vi "get write location linear fit.vi"(7 "use line and frame numbers":bool, 9 "xyz order":bool, 10 "current volume":T1={"min x"=-1638, "deltaX"=41.0, "num x"=79, "max x"=1601, "min y"=-1638, "deltaY"=41.0, "num y"=80, "max y"=1642, "num z"=30, "num voxels"=189600, "voxels read"=0, "volume num"=0}, 11 "line":T2) -> (3 "3D write locations":u32[](array[numeric]))   [LabVIEW 2010]
uses:
  line_info.ctl
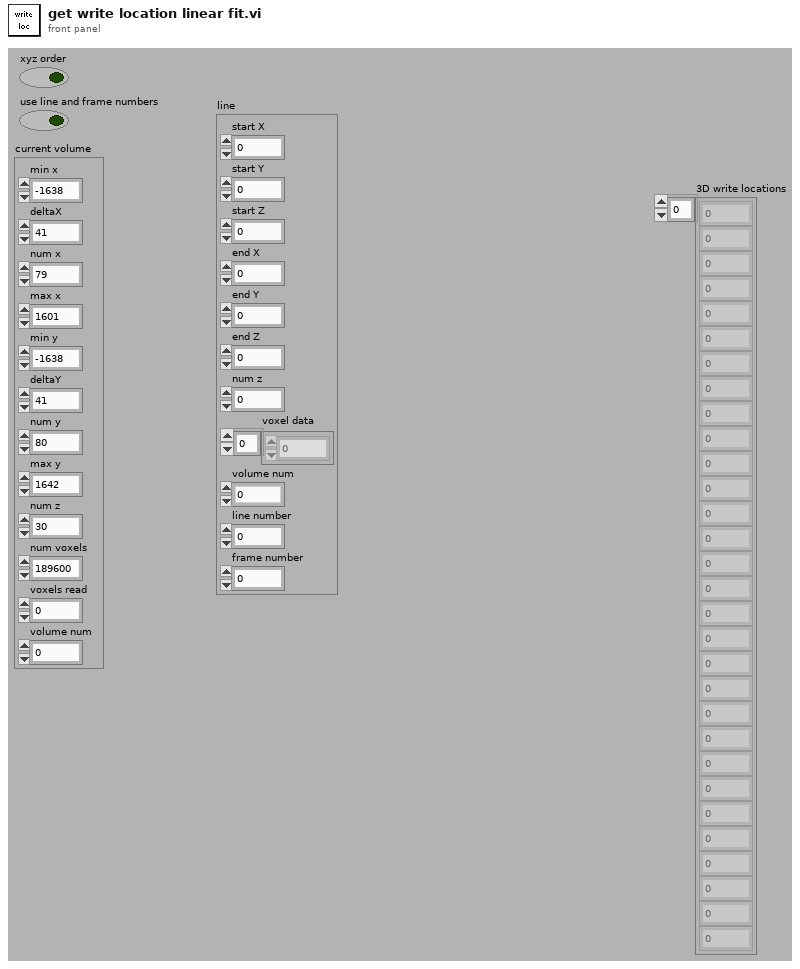
[diagram p1: front panel]
types:
  T1 = cluster{"min x":i16, "deltaX":dbl, "num x":u32, "max x":i16, "min y":i16, "deltaY":dbl, "num y":u32, "max y":i16, "num z":u32, "num voxels":u32, "voxels read":u32, "volume num":u32}
  T2 = typedef "line_info.ctl" = cluster{"start X":i16, "start Y":i16, "start Z":i16, "end X":i16, "end Y":i16, "end Z":i16, "num z":u8, "voxel data":u32[], "volume num":u32, "line number":u16, "frame number":u16}
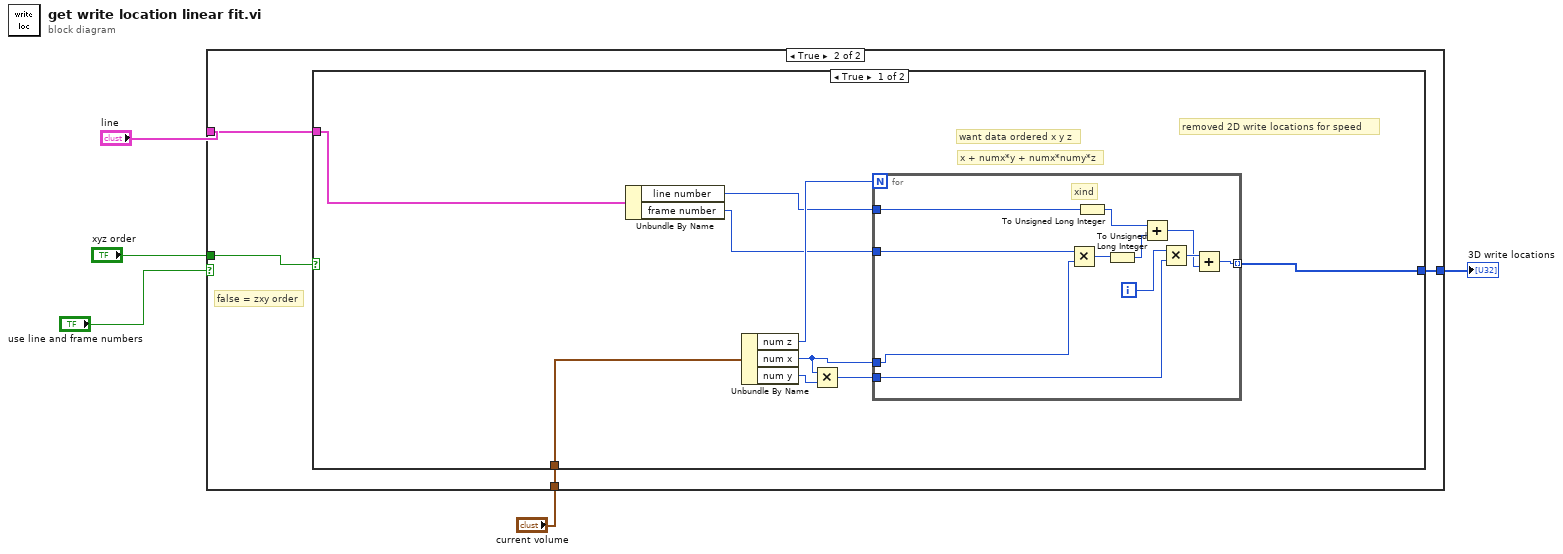
[diagram p0: block diagram]
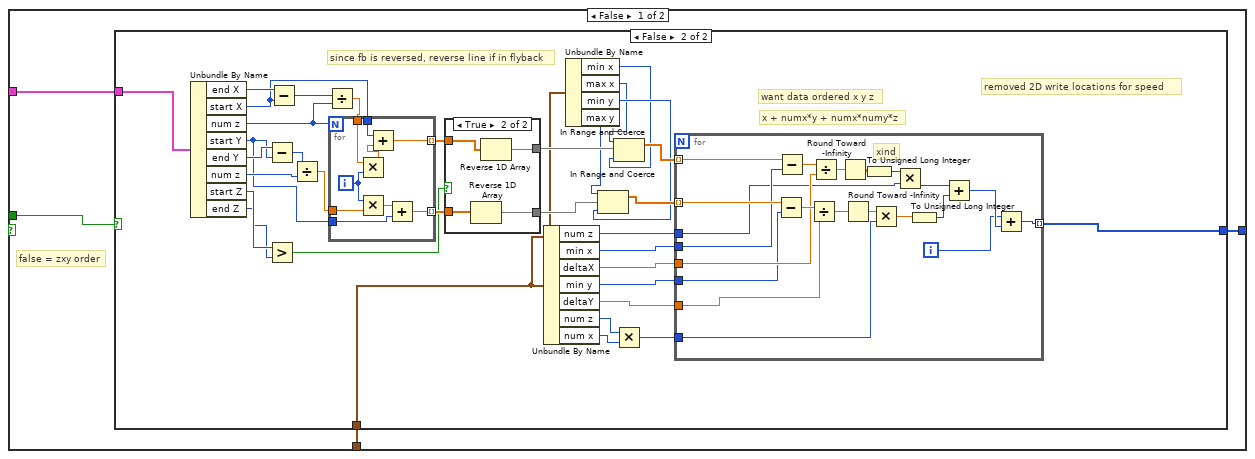
[diagram p2: hidden frame]
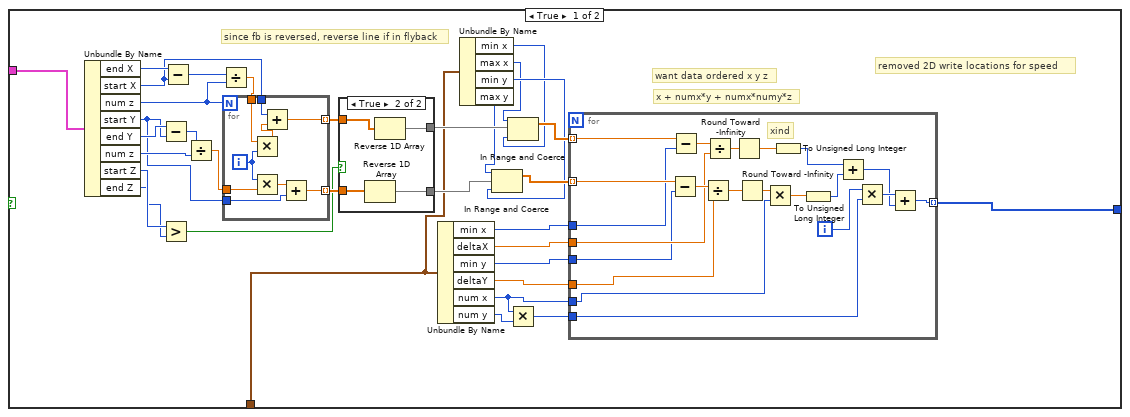
[diagram p3: hidden frame]
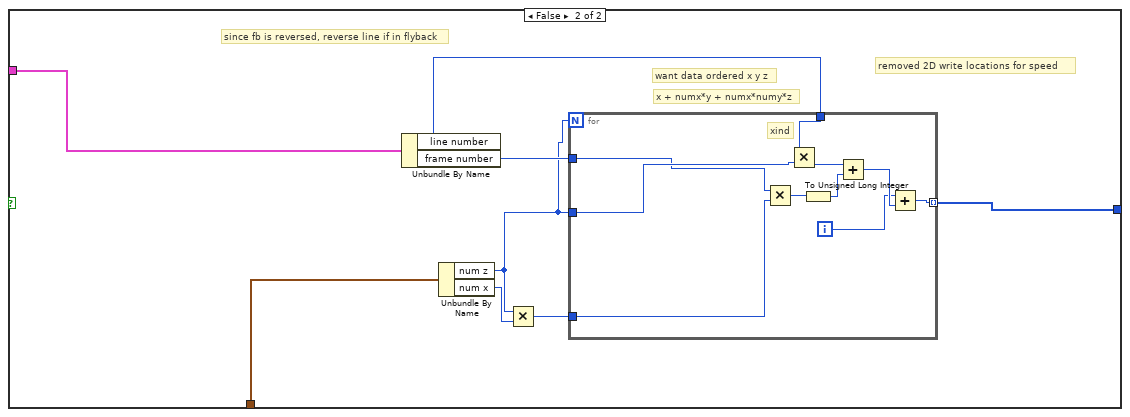
[diagram p6: hidden frame]
diagram:
  n1 = case shown="True" "use line and frame numbers" {
    tunnel: "line" -> [w9 w152]
    tunnel: "xyz order" -> [w8 w151]
    tunnel: "current volume" -> [w7 w150]
    tunnel: [w6 w149] -> w2
    frame False {
      # "false = zxy order"
      n2 = case shown="False" w8 {
        tunnel: w9 -> [w42 w112]
        tunnel: w7 -> [w11 w81]
        tunnel: [w10 w80] -> w6
        frame True {
          # "removed 2D write locations for speed"
          # "x + numx*y + numx*numy*z"
          # "want data ordered x y z"
          # "since fb is reversed, reverse line if in flyback"
          n3 = Unbundle By Name(w42) -> ("end X"=w41:i16, "start X"=w38:i16, "num z"=w37:u8, "start Y"=w12:i16, "end Y"=w13:i16, "num z"=w35:u8, "start Z"=w33:i16, "end Z"=w32:i16)
          n4 = Subtract(x=w13, y=w12) -> (x-y=w36:i16)
          n5 = Greater?(x=w33, y=w32) -> (0:w16:bool)
          n6 = Subtract(x=w41, y=w38) -> (x-y=w40:i16)
          n7 = Divide(x=w36, y=w35) -> (x/y=w34:dbl)
          n8 = Divide(x=w40, y=w37) -> (x/y=w39:dbl)
          n9 = for {
            N: w37 -> [_]
            tunnel: w39 -> [w78]
            tunnel: w38 -> [w77]
            tunnel: [w75] -> w30 mode=indexing
            tunnel: w34 -> [w73]
            tunnel: w12 -> [w71]
            tunnel: [w70] -> w31 mode=indexing
            i -> [w74]
            n10 = Multiply(x=w78, y=w74) -> (x*y=w76:dbl)
            n11 = Multiply(x=w74, y=w73) -> (x*y=w72:dbl)
            n12 = Add(x=w77, y=w76) -> (x+y=w75:dbl)
            n13 = Add(x=w72, y=w71) -> (x+y=w70:dbl)
          }
          n14 = case shown="True" w16 {
            tunnel: w31 -> [w64 w67]
            tunnel: w30 -> [w65 w69]
            tunnel: [w65 w68] -> w20
            tunnel: [w64 w66] -> w29
            frame False {
            }
            frame True {
              n15 = Reverse 1D Array(array=w67) -> (reversed array=w66:dbl[])
              n16 = Reverse 1D Array(array=w69) -> (reversed array=w68:dbl[])
            }
          }
          n17 = Unbundle By Name(w11) -> ("min x"=w28:i16, "deltaX"=w27:dbl, "min y"=w26:i16, "deltaY"=w25:dbl, "num x"=w24:u32, "num y"=w23:u32)
          n18 = Unbundle By Name(w11) -> ("min x"=w14:i16, "max x"=w15:i16, "min y"=w17:i16, "max y"=w18:i16)
          n19 = In Range and Coerce(upper limit=w18, x=w29, lower limit=w17) -> (coerced(x)=w19:dbl[])  [unwired: 1 out]
          n20 = In Range and Coerce(upper limit=w15, x=w20, lower limit=w14) -> (coerced(x)=w21:dbl[])  [unwired: 1 out]
          n21 = Multiply(x=w24, y=w23) -> (x*y=w22:u32)
          n22 = for {
            tunnel: [w51] -> w10 mode=indexing
            tunnel: w21 -> [w54] mode=indexing
            tunnel: w19 -> [w53] mode=indexing
            tunnel: w28 -> [w50]
            tunnel: w27 -> [w49]
            tunnel: w26 -> [w48]
            tunnel: w25 -> [w47]
            tunnel: w24 -> [w46]
            tunnel: w22 -> [w45]
            i -> [w44]
            # "xind"
            n23 = Subtract(x=w53, y=w48) -> (x-y=w61:dbl)
            n24 = Subtract(x=w54, y=w50) -> (x-y=w63:dbl)
            n25 = Divide(x=w61, y=w47) -> (x/y=w60:dbl)
            n26 = Divide(x=w63, y=w49) -> (x/y=w62:dbl)
            n27 = Round Toward -Infinity(1:w62) -> (0:w58:dbl)
            n28 = Round Toward -Infinity(1:w60) -> (0:w59:dbl)
            n29 = Multiply(x=w59, y=w46) -> (x*y=w57:dbl)
            n30 = To Unsigned Long Integer(number=w58) -> (unsigned 32bit integer=w56:u32)
            n31 = To Unsigned Long Integer(number=w57) -> (unsigned 32bit integer=w55:u32)
            n32 = Add(x=w56, y=w55) -> (x+y=w43:u32)
            n33 = Multiply(x=w44, y=w45) -> (x*y=w52:u32)
            n34 = Add(x=w52, y=w43) -> (x+y=w51:u32)
          }
        }
        frame False {
          # "removed 2D write locations for speed"
          # "x + numx*y + numx*numy*z"
          # "want data ordered x y z"
          # "since fb is reversed, reverse line if in flyback"
          n35 = Unbundle By Name(w112) -> ("end X"=w111:i16, "start X"=w108:i16, "num z"=w107:u8, "start Y"=w82:i16, "end Y"=w83:i16, "num z"=w105:u8, "start Z"=w103:i16, "end Z"=w102:i16)
          n36 = Subtract(x=w83, y=w82) -> (x-y=w106:i16)
          n37 = Greater?(x=w103, y=w102) -> (0:w86:bool)
          n38 = Subtract(x=w111, y=w108) -> (x-y=w110:i16)
          n39 = Divide(x=w106, y=w105) -> (x/y=w104:dbl)
          n40 = Divide(x=w110, y=w107) -> (x/y=w109:dbl)
          n41 = for {
            N: w107 -> [_]
            tunnel: w109 -> [w148]
            tunnel: w108 -> [w147]
            tunnel: [w145] -> w100 mode=indexing
            tunnel: w104 -> [w143]
            tunnel: w82 -> [w141]
            tunnel: [w140] -> w101 mode=indexing
            i -> [w144]
            n42 = Multiply(x=w148, y=w144) -> (x*y=w146:dbl)
            n43 = Multiply(x=w144, y=w143) -> (x*y=w142:dbl)
            n44 = Add(x=w147, y=w146) -> (x+y=w145:dbl)
            n45 = Add(x=w142, y=w141) -> (x+y=w140:dbl)
          }
          n46 = case shown="True" w86 {
            tunnel: w101 -> [w134 w137]
            tunnel: w100 -> [w135 w139]
            tunnel: [w135 w138] -> w90
            tunnel: [w134 w136] -> w99
            frame False {
            }
            frame True {
              n47 = Reverse 1D Array(array=w137) -> (reversed array=w136:dbl[])
              n48 = Reverse 1D Array(array=w139) -> (reversed array=w138:dbl[])
            }
          }
          n49 = Unbundle By Name(w81) -> ("num z"=w79:u32, "min x"=w98:i16, "deltaX"=w97:dbl, "min y"=w96:i16, "deltaY"=w95:dbl, "num z"=w94:u32, "num x"=w93:u32)
          n50 = Unbundle By Name(w81) -> ("min x"=w84:i16, "max x"=w85:i16, "min y"=w87:i16, "max y"=w88:i16)
          n51 = In Range and Coerce(upper limit=w88, x=w99, lower limit=w87) -> (coerced(x)=w89:dbl[])  [unwired: 1 out]
          n52 = In Range and Coerce(upper limit=w85, x=w90, lower limit=w84) -> (coerced(x)=w91:dbl[])  [unwired: 1 out]
          n53 = Multiply(x=w94, y=w93) -> (x*y=w92:u32)
          n54 = for {
            tunnel: [w122] -> w80 mode=indexing
            tunnel: w91 -> [w124] mode=indexing
            tunnel: w89 -> [w123] mode=indexing
            tunnel: w98 -> [w121]
            tunnel: w97 -> [w120]
            tunnel: w96 -> [w119]
            tunnel: w95 -> [w118]
            tunnel: w92 -> [w114]
            tunnel: w79 -> [w115]
            i -> [w113]
            # "xind"
            n55 = Subtract(x=w123, y=w119) -> (x-y=w131:dbl)
            n56 = Subtract(x=w124, y=w121) -> (x-y=w133:dbl)
            n57 = Divide(x=w131, y=w118) -> (x/y=w130:dbl)
            n58 = Divide(x=w133, y=w120) -> (x/y=w132:dbl)
            n59 = Round Toward -Infinity(1:w132) -> (0:w128:dbl)
            n60 = Round Toward -Infinity(1:w130) -> (0:w129:dbl)
            n61 = To Unsigned Long Integer(number=w128) -> (unsigned 32bit integer=w126:u32)
            n62 = Multiply(x=w129, y=w114) -> (x*y=w127:dbl)
            n63 = Multiply(x=w126, y=w115) -> (x*y=w116:u32)
            n64 = To Unsigned Long Integer(number=w127) -> (unsigned 32bit integer=w125:u32)
            n65 = Add(x=w116, y=w125) -> (x+y=w117:u32)
            n66 = Add(x=w113, y=w117) -> (x+y=w122:u32)
          }
        }
      }
    }
    frame True {
      # "false = zxy order"
      n67 = case shown="True" w151 {
        tunnel: w152 -> [w155 w180]
        tunnel: w150 -> [w158 w177]
        tunnel: [w157 w176] -> w149
        frame True {
          # "removed 2D write locations for speed"
          # "x + numx*y + numx*numy*z"
          # "want data ordered x y z"
          n68 = Unbundle By Name(w155) -> ("line number"=w154:u16, "frame number"=w153:u16)
          n69 = Unbundle By Name(w158) -> ("num z"=w156:u32, "num x"=w161:u32, "num y"=w160:u32)
          n70 = Multiply(x=w161, y=w160) -> (x*y=w159:u32)
          n71 = for {
            N: w156 -> [_]
            tunnel: [w168] -> w157 mode=indexing
            tunnel: w161 -> [w167]
            tunnel: w159 -> [w166]
            tunnel: w154 -> [w163]
            tunnel: w153 -> [w162]
            i -> [w165]
            # "xind"
            n72 = Multiply(x=w162, y=w167) -> (x*y=w172:u32)
            n73 = To Unsigned Long Integer(number=w163) -> (unsigned 32bit integer=w171:u32)
            n74 = To Unsigned Long Integer(number=w172) -> (unsigned 32bit integer=w170:u32)
            n75 = Add(x=w171, y=w170) -> (x+y=w164:u32)
            n76 = Multiply(x=w165, y=w166) -> (x*y=w169:u32)
            n77 = Add(x=w169, y=w164) -> (x+y=w168:u32)
          }
        }
        frame False {
          # "removed 2D write locations for speed"
          # "x + numx*y + numx*numy*z"
          # "want data ordered x y z"
          # "since fb is reversed, reverse line if in flyback"
          n78 = Unbundle By Name(w180) -> ("line number"=w175:u16, "frame number"=w174:u16)
          n79 = Unbundle By Name(w177) -> ("num z"=w173:u32, "num x"=w179:u32)
          n80 = Multiply(x=w173, y=w179) -> (x*y=w178:u32)
          n81 = for {
            N: w173 -> [_]
            tunnel: [w188] -> w176 mode=indexing
            tunnel: w178 -> [w184]
            tunnel: w173 -> [w185]
            tunnel: w175 -> [w182]
            tunnel: w174 -> [w181]
            i -> [w183]
            # "xind"
            n82 = Multiply(x=w181, y=w184) -> (x*y=w190:u32)
            n83 = Multiply(x=w182, y=w185) -> (x*y=w186:u32)
            n84 = To Unsigned Long Integer(number=w190) -> (unsigned 32bit integer=w189:u32)
            n85 = Add(x=w186, y=w189) -> (x+y=w187:u32)
            n86 = Add(x=w183, y=w187) -> (x+y=w188:u32)
          }
        }
      }
    }
  }
  "3D write locations" <- w2
